vi "SaveAcquiredImageBMP.vi"(8 "error in":errorcluster, 10 "File Name":string, 11 "Folder Path":string) -> (0 "error out":errorcluster, 4 "return":i32)   [LabVIEW 2015]
uses:
  [Global] Image.vi
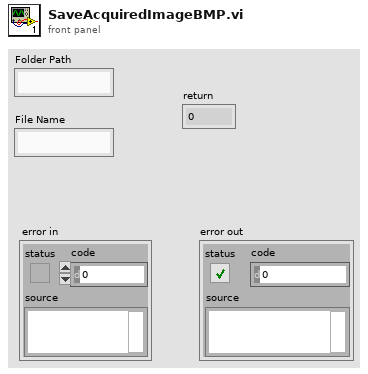
[diagram p1: front panel]
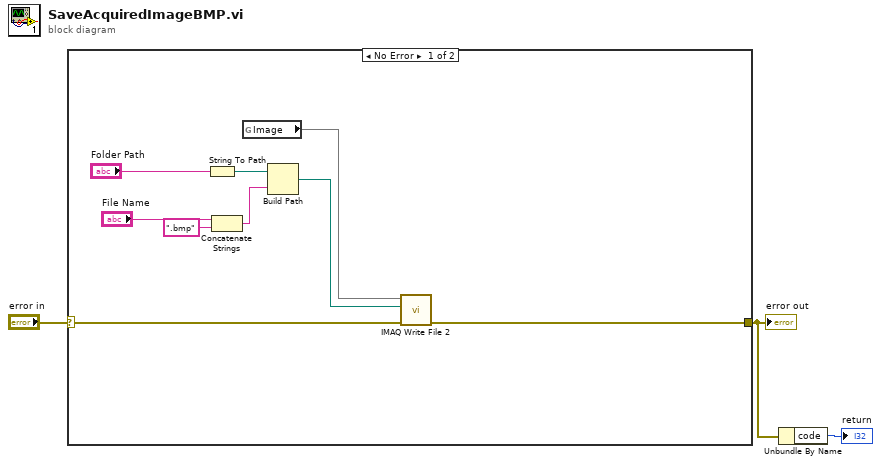
[diagram p0: block diagram]
diagram:
  n1 = case shown="No Error" "error in" {
    selector: "error in" -> [w12 w13]
    tunnel: [w11 w13] -> w1
    frame No Error {
      n2 = String To Path(string="Folder Path") -> (path=w10:path)
      n3 = Concatenate Strings("File Name", ".bmp" ("string")) -> (w8:string)
      n4 = global read "[Global] Image.vi" "Image"() -> (w4)
      n5 = Build Path(base path=w10, name or relative path=w8) -> (appended path=w5:path)
      n6 = call-poly "IMAQ Write File 2"("error in (no error)"=w12, "File Path"=w5, "Image"=w4) -> ("error out"=w11:errorcluster)  [unwired: 7 in, 1 out]
    }
    frame Error {
    }
  }
  "error out" <- w1
  n7 = Unbundle By Name(w1) -> ("code"=→"return":i32)
